vi "fn Lumencor DLL2b.vi"(8 "error in (no error)":errorcluster) -> (0 "error out":errorcluster, 3 "function return":i32)   [LabVIEW 2017, in "LumencorDLLDbg64.lvlib"]
doc: "LUMENCORDLL2B_API int fnLumencorDLL2b(void);"
uses:
  LumencorDLLDbg64.lvlib
  LumencorDLLDbg64.dll
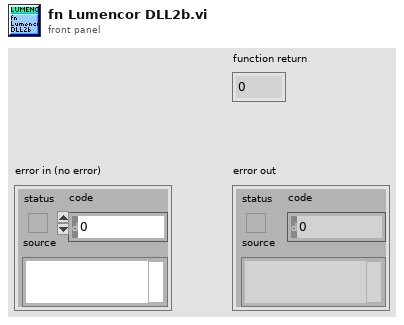
[diagram p1: front panel]
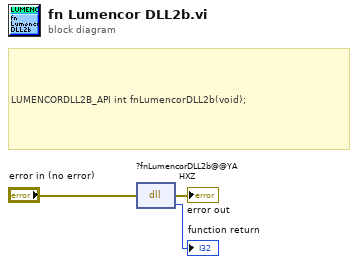
[diagram p0: block diagram]
diagram:
  # "LUMENCORDLL2B_API int fnLumencorDLL2b(void);"
  n1 = dll-call lib="Q:/GIT -- Lumencor DLL4/LabVIEW Library (64bit)/LumencorDLLDbg64.*" fn="?fnLumencorDLL2b@@YAHXZ"(error in="error in (no error)") -> (error out=→"error out":errorcluster, →"function return":i32)  [unwired: 2 in, 1 out]
